vi "Generate_Argument_List.vi"(1 "Command":string) -> (0 "Argument List":string[](array[string]))   [LabVIEW 2011]
doc: "Generates a default argument list for a given command."
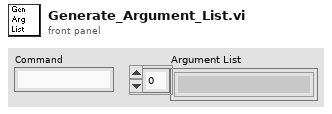
[diagram p1: front panel]
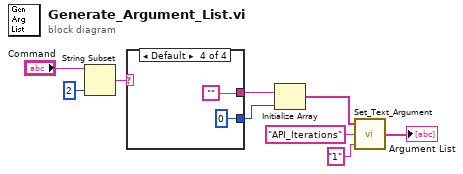
[diagram p0: block diagram]
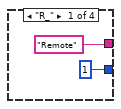
[diagram p2: hidden frame]
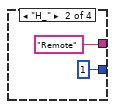
[diagram p3: hidden frame]
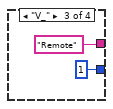
[diagram p4: hidden frame]
diagram:
  n1 = String Subset(string="Command", length (rest)=2 ("length (rest)")) -> (substring=w9:string)  [unwired: 1 out]
  n2 = case shown="Default" w9 {
    tunnel: ["Remote" ("element") "Remote" ("element") "Remote" ("element") ""] -> w7
    tunnel: [1 ("dimension size") 1 ("dimension size") 1 ("dimension size") 0 ("dimension size")] -> w6
    frame "R_" {
    }
    frame "H_" {
    }
    frame "V_" {
    }
    frame Default {
    }
  }
  n3 = Initialize Array(w7, w6) -> (w5:string[])
  n4 = call "Set_Text_Argument.vi"("Text"="1", "Argument"="API_Iterations", "Argument List In"=w5) -> ("Argument List Out"=→"Argument List":string[])
